vi "oax_gsSnd Write Wave File+.vi"(4 "stereo 16-bit":i16[][](array[numeric]), 5 "mono 16-bit":i16[](array[numeric]), 6 "stereo 8-bit":u8[][](array[numeric]), 7 "mono 8-bit":u8[](array[numeric]), 8 "error in (no error)":errorcluster, 10 "sound format":T1, 11 "wave file path":path) -> (0 "error out":errorcluster, 3 "wave file path out":path)   [LabVIEW 2017]
doc: "This vi writes sound data to a PC waveform audio file which can be later read by Snd Read Wave File or other applications."
uses:
  <vilib>/addons/Sound and Vibration/Order Analysis/Example Support/Demo VI/subVIs/oax_gsSound Format+.ctl
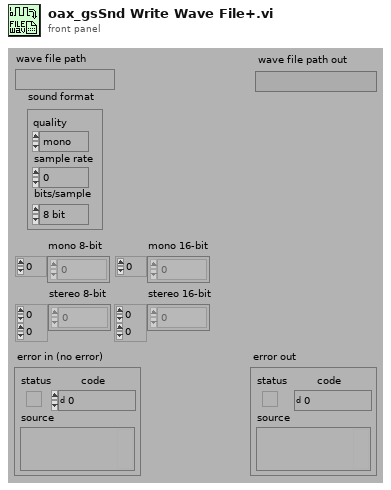
[diagram p1: front panel]
types:
  T1 = typedef "oax_gsSound Format+.ctl" = cluster{"quality":enum16{"mono", "stereo"}, "sample rate":u32, "bits/sample":enum16{"8 bit", "16 bit"}}
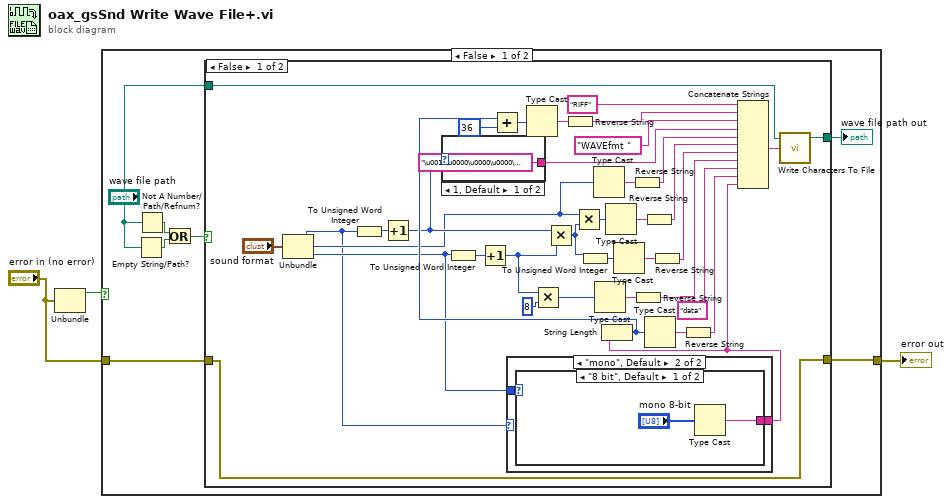
[diagram p0: block diagram]
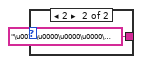
[diagram p2: hidden frame]
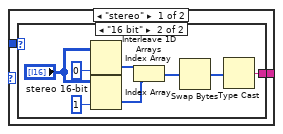
[diagram p3: hidden frame]
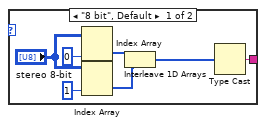
[diagram p4: hidden frame]
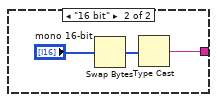
[diagram p5: hidden frame]
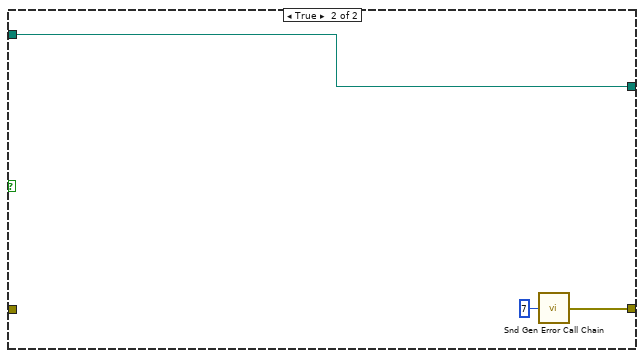
[diagram p6: hidden frame]
diagram:
  n1 = Unbundle("error in (no error)") -> ("status"=w1:bool)  [unwired: 2 out]
  n2 = case shown="False" w1 {
    tunnel: [w4 w77] -> w3
    tunnel: "error in (no error)" -> [w5 w77]
    frame False {
      n3 = Empty String/Path?(string/path="wave file path") -> (empty?=w9:bool)
      n4 = Not A Number/Path/Refnum?(number/path/refnum="wave file path") -> (NaN/Path/Refnum?=w10:bool)
      n5 = Or(x=w10, y=w9) -> (x .or. y?=w8:bool)
      n6 = case shown="False" w8 {
        tunnel: "wave file path" -> [w25 w76]
        tunnel: [w24 w76] -> w6
        tunnel: [w23 w74] -> w4
        tunnel: w5 -> [w23 _]
        frame False {
          n7 = Unbundle("sound format") -> ("quality"=w11:enum16{"mono", "stereo"}, "sample rate"=w17:u32, "bits/sample"=w12:enum16{"8 bit", "16 bit"})
          n8 = To Unsigned Word Integer(number=w11) -> (unsigned 16bit integer=w19:u16)
          n9 = Increment(x=w19) -> (x+1=w18:u16)
          n10 = case shown="1, Default" w18 {
            tunnel: ["\u0010\u0000\u0000\u0000\u0001\u0000\u0001\u0000" "\u0010\u0000\u0000\u0000\u0001\u0000\u0002\u0000"] -> w26
            frame 1, Default {
            }
            frame 2 {
            }
          }
          n11 = To Unsigned Word Integer(number=w12) -> (unsigned 16bit integer=w16:u16)
          n12 = Increment(x=w16) -> (x+1=w13:u16)
          n13 = case shown="\"mono\", Default" w11 {
            tunnel: [w51 w68] -> w28
            tunnel: w12 -> [w50 w67]
            frame "stereo" {
              n14 = case shown="\"16 bit\"" w50 {
                tunnel: [w52 w59] -> w51
                frame "8 bit", Default {
                  n15 = Index Array(array="stereo 8-bit", index (col)=0) -> (element=w55:u8[])  [unwired: 1 in]
                  n16 = Index Array(array="stereo 8-bit", index (col)=1) -> (element=w54:u8[])  [unwired: 1 in]
                  n17 = Interleave 1D Arrays(w55, w54) -> (w53:u8[])
                  n18 = Type Cast(x=w53) -> (*(type *) &x=w52:string)  [unwired: 1 in]
                }
                frame "16 bit" {
                  n19 = Index Array(array="stereo 16-bit", index (col)=0) -> (element=w64:i16[])  [unwired: 1 in]
                  n20 = Index Array(array="stereo 16-bit", index (col)=1) -> (element=w63:i16[])  [unwired: 1 in]
                  n21 = Interleave 1D Arrays(w64, w63) -> (w61:i16[])
                  n22 = Swap Bytes(anything=w61) -> (byte swapped=w60:i16[])
                  n23 = Type Cast(x=w60) -> (*(type *) &x=w59:string)  [unwired: 1 in]
                }
              }
            }
            frame "mono", Default {
              n24 = case shown="\"8 bit\", Default" w67 {
                tunnel: [w69 w71] -> w68
                frame "8 bit", Default {
                  n25 = Type Cast(x="mono 8-bit") -> (*(type *) &x=w69:string)  [unwired: 1 in]
                }
                frame "16 bit" {
                  n26 = Swap Bytes(anything="mono 16-bit") -> (byte swapped=w73:i16[])
                  n27 = Type Cast(x=w73) -> (*(type *) &x=w71:string)  [unwired: 1 in]
                }
              }
            }
          }
          n28 = Multiply(x=w13, y=u16 8) -> (x*y=w14:u16)
          n29 = Multiply(x=w18, y=w13) -> (x*y=w33:u16)
          n30 = Multiply(x=w17, y=w33) -> (x*y=w35:u32)
          n31 = To Unsigned Word Integer(number=w33) -> (unsigned 16bit integer=w32:u16)
          n32 = Type Cast(x=w17) -> (*(type *) &x=w39:string)  [unwired: 1 in]
          n33 = Type Cast(x=w14) -> (*(type *) &x=w22:string)  [unwired: 1 in]
          n34 = String Length(string=w28) -> (length=w40:i32)
          n35 = Add(x=w40, y=36) -> (x+y=w42:i32)
          n36 = Type Cast(x=w42) -> (*(type *) &x=w44:string)  [unwired: 1 in]
          n37 = Reverse String(1:w44) -> (0:w41:string)
          n38 = Type Cast(x=w35) -> (*(type *) &x=w37:string)  [unwired: 1 in]
          n39 = Type Cast(x=w32) -> (*(type *) &x=w34:string)  [unwired: 1 in]
          n40 = Reverse String(1:w39) -> (0:w38:string)
          n41 = Reverse String(1:w22) -> (0:w21:string)
          n42 = Reverse String(1:w37) -> (0:w36:string)
          n43 = Type Cast(x=w40) -> (*(type *) &x=w45:string)  [unwired: 1 in]
          n44 = Reverse String(1:w34) -> (0:w31:string)
          n45 = Reverse String(1:w45) -> (0:w29:string)
          n46 = Concatenate Strings("RIFF", w41, "WAVEfmt ", w26, w38, w36, w31, w21, "data", w29, w28) -> (w27:string)
          n47 = call <vilib>:"Write Characters To File.vi"("character string"=w27, "file path (dialog if empty)"=w25) -> ("new file path (Not A Path if cancelled)"=w24:path)  [unwired: 3 in]
        }
        frame True {
          n48 = call <vilib>:"Snd Gen Error Call Chain.vi"("error code"=7) -> ("error out"=w74:errorcluster)
        }
      }
      "wave file path out" <- w6
    }
    frame True {
    }
  }
  "error out" <- w3
